vi "判断数组大小并截取子集.vi"(10 "数组":string[](array[string]), 11 "截取数组大小":dbl) -> (2 "输出数组":string[](array[string]))   [LabVIEW 2019]
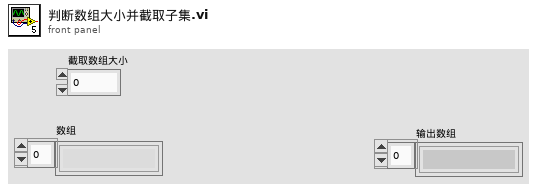
[diagram p1: front panel]
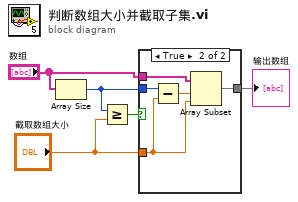
[diagram p0: block diagram]
diagram:
  n1 = Array Size(array="数组") -> (size(s)=w2:i32)
  n2 = Greater Or Equal?(x=w2, y="截取数组大小") -> (x >= y?=w4:bool)
  n3 = case shown="True" w4 {
    tunnel: "数组" -> [w6 w11]
    tunnel: "截取数组大小" -> [_ w9]
    tunnel: w2 -> [_ w8]
    tunnel: [w6 w7] -> w1
    frame False {
    }
    frame True {
      n4 = Subtract(x=w8, y=w9) -> (x-y=w10:dbl)
      n5 = Array Subset(array=w11, index=w10, length=w9) -> (w7:string[])
    }
  }
  "输出数组" <- w1
